vi "Uarm Initialize.vi"(8 "error in":errorcluster, 10 "full read buffer in":string, 11 "Machine In":refnum<visa-resource-name>) -> (0 "error out":errorcluster, 2 "full read buffer out":string, 3 "Machine Out":refnum<visa-resource-name>)   [LabVIEW 2017]
panel:
  out "read buffer":string
  out "G-Code String":string
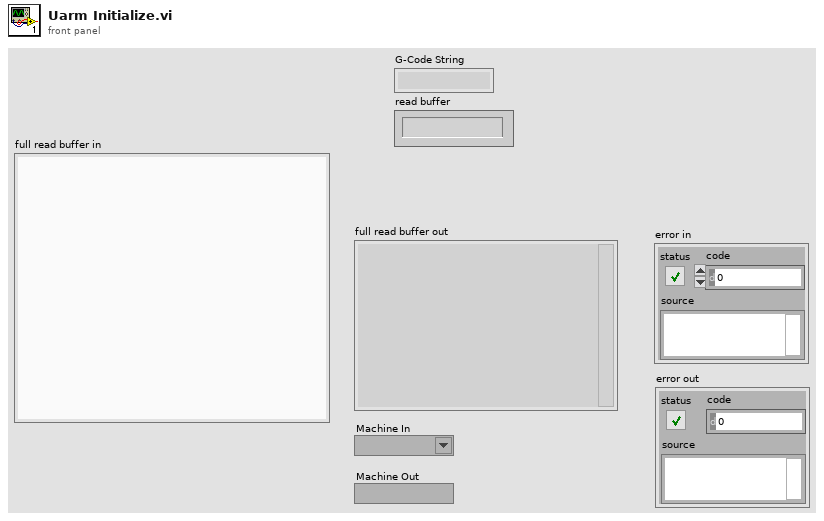
[diagram p1: front panel]
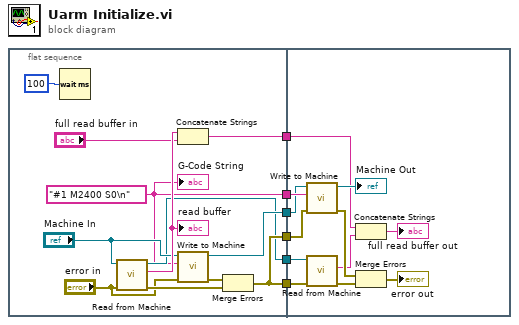
[diagram p0: block diagram]
diagram:
  n1 = flat-sequence {
    tunnel: [w15] -> w6
    tunnel: [w15] -> w5
    tunnel: [w9] -> w4
    tunnel: [w11] -> w3
    tunnel: [w10] -> w2
    tunnel: [w8] -> w1
    tunnel: w6 -> [w30]
    tunnel: w5 -> [w29]
    tunnel: w4 -> [w25]
    tunnel: w3 -> [w24]
    tunnel: w2 -> [w23]
    tunnel: w1 -> [w20]
    frame #0 {
      w9 = "#1 M2400 S0\n"
      n2 = Wait (ms)(milliseconds to wait=u32 100) -> ()  [unwired: 1 out]
      n3 = call "Read from Machine.vi"("error in (no error)"="error in", "Machine In"="Machine In") -> ("error out"=w16:errorcluster, "read buffer"=w14:string, "Machine Out"=w10:refnum<visa-resource-name>)  [unwired: 7 in]
      "read buffer" <- w14
      n4 = Concatenate Strings(w14, "full read buffer in") -> (w8:string)
      n5 = call "Write to Machine .vi"("error in (no error)"="error in", "G-Code String In"=w9, "Machine In"="Machine In") -> ("error out"=w17:errorcluster, "Machine Out"=w11:refnum<visa-resource-name>)  [unwired: 7 in]
      n6 = Merge Errors(w17, w16) -> (w15:errorcluster)
      "G-Code String" <- w9
    }
    frame #1 {
      n7 = call "Write to Machine .vi"("error in (no error)"=w30, "G-Code String In"=w25, "Machine In"=w24) -> ("error out"=w27:errorcluster, "Machine Out"=→"Machine Out":refnum<visa-resource-name>)  [unwired: 7 in]
      n8 = call "Read from Machine.vi"("error in (no error)"=w29, "Machine In"=w23) -> ("error out"=w26:errorcluster, "read buffer"=w21:string)  [unwired: 7 in, 1 out]
      n9 = Concatenate Strings(w20, w21) -> (→"full read buffer out":string)
      n10 = Merge Errors(w27, w26) -> (→"error out":errorcluster)
    }
  }
